vi "Create Math Operation.vi"(6 "Custom Math Operation Formula (\"(((RES - 10e3)/10e3)*100)\")":string="(((RES - 10e3)/10e3)*100)", 8 "error in (no error)":errorcluster, 9 "Custom Math Operation Unit (\"%\")":string="%", 10 "Custom Math Operation Name (\"PCT_DEV\")":string="PCT_DEV", 11 "VISA resource name":refnum<visa-resource-name>) -> (0 "error out":errorcluster, 3 "VISA resource name out":refnum<visa-resource-name>)   [LabVIEW 2019, in "Keithley 24XX.lvlib"]
doc: "Creates a custom math operation that can then be used with Configure Math."
uses:
  Keithley 24XX.lvlib
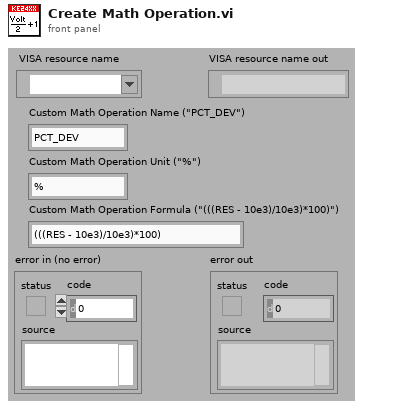
[diagram p1: front panel]
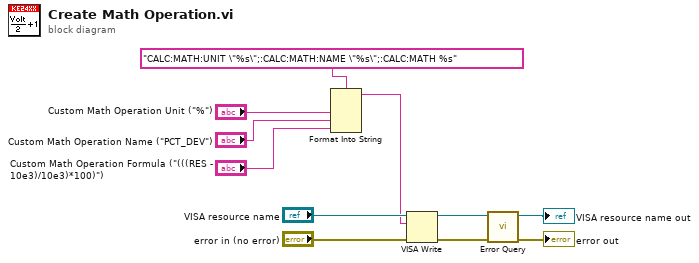
[diagram p0: block diagram]
diagram:
  n1 = Format Into String(format string="CALC:MATH:UNIT \"%s\";:CALC:MATH:NAME \"%s\";:CALC:MATH %s", "Custom Math Operation Unit (\"%\")", "Custom Math Operation Name (\"PCT_DEV\")", "Custom Math Operation Formula (\"(((RES - 10e3)/10e3)*100)\")") -> (resulting string=w3:string)  [unwired: 2 in, 1 out]
  n2 = VISA Write(VISA resource name="VISA resource name", write buffer=w3, error in (no error)="error in (no error)") -> (VISA resource name out=w9:refnum<visa-resource-name>, error out=w6:errorcluster)  [unwired: 1 out]
  n3 = call "Error Query.vi"("error in (no error)"=w6, "VISA resource name"=w9) -> ("error out"=→"error out":errorcluster, "VISA resource name out"=→"VISA resource name out":refnum<visa-resource-name>)  [unwired: 6 in, 2 out]
